vi "Parse.Paths.Parse.vi"() -> ()   [LabVIEW 2020, in "Parse.Paths.lvclass"]
uses:
  Parse.Paths.lvclass
  PathCommands/PathCommands.lvclass
  PathTokenizer/PathTokenizer.lvclass
  PathTokenizer/PathTokenizer.lvclass/PathTokenizer.ctl
  PathCommands.LineTo/PathCommands.LineTo.lvclass
  C:/Users/Albro/Documents/GitHub/AFM-Lithography/lvsrc/Classes/Parse/PathCommands/PathCommands.lvclass
  PathCommands.CurveTo/PathCommands.CurveTo.lvclass
  PathCommands.Moveto/PathCommands.MoveTo.lvclass
  PathCommands.ClosePath/PathCommands.ClosePath.lvclass
panel:
  out "Array":refnum<class "PathCommands.lvclass">[](array[class])
  in  "Path Input":string
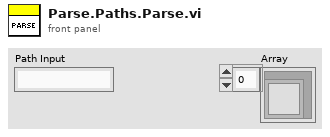
[diagram p1: front panel]
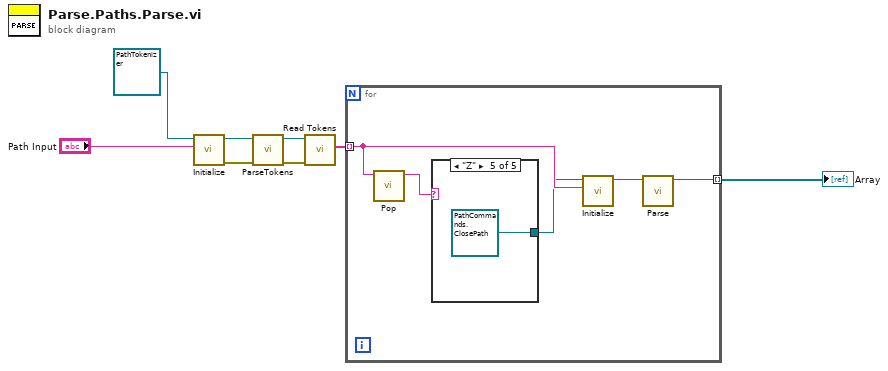
[diagram p0: block diagram]
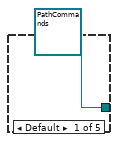
[diagram p2: hidden frame]
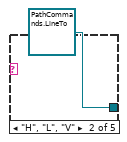
[diagram p3: hidden frame]
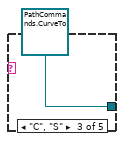
[diagram p4: hidden frame]
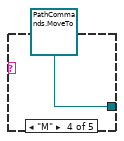
[diagram p5: hidden frame]
diagram:
  n1 = call "Initialize.vi"("Path Command Text"="Path Input", "PathTokenizer in"=refnum<class "PathTokenizer.lvclass"> refnum) -> ("error out"=w3:errorcluster, "PathTokenizer out"=w6:refnum<class "PathTokenizer.lvclass">)  [unwired: 8 in]
  n2 = call "ParseTokens.vi"("error in (no error)"=w3, "PathTokenizer in"=w6) -> ("error out"=w4:errorcluster, "PathTokenizer out"=w5:refnum<class "PathTokenizer.lvclass">)  [unwired: 8 in]
  n3 = call "Read Tokens.vi"("error in (no error)"=w4, "PathTokenizer in"=w5) -> ("Tokens"=w2:string[])  [unwired: 7 in, 2 out]
  n4 = for {
    tunnel: w2 -> [w12] mode=indexing
    tunnel: [w9] -> w1 mode=indexing
    n5 = call "Pop.vi"("Command Text"=w12) -> ("Command Type"=w13:string)  [unwired: 9 in, 1 out]
    n6 = case shown="\"Z\"" w13 {
      tunnel: [refnum<class "PathCommands.lvclass"> refnum ("PathCommands.lvclass") refnum<class "PathCommands.LineTo.lvclass"> refnum ("PathCommands.LineTo.lvclass") refnum<class "PathCommands.CurveTo.lvclass"> refnum ("PathCommands.CurveTo.lvclass") refnum<class "PathCommands.MoveTo.lvclass"> refnum ("PathCommands.MoveTo.lvclass") refnum<class "PathCommands.ClosePath.lvclass"> refnum ("PathCommands.ClosePath.lvclass")] -> w10
      frame Default {
      }
      frame "H", "L", "V" {
      }
      frame "C", "S" {
      }
      frame "M" {
      }
      frame "Z" {
      }
    }
    n7 = call-dynamic "Initialize.vi"("CommandText"=w12, "PathCommands in"=w10) -> ("PathCommands out"=w11:refnum<class "PathCommands.lvclass">)  [unwired: 8 in, 1 out]
    n8 = call-dynamic "Parse.vi"("PathCommands in"=w11) -> ("PathCommands out"=w9:refnum<class "PathCommands.lvclass">)  [unwired: 9 in, 1 out]
  }
  "Array" <- w1
